vi "KI -Set Integral gain.vi"(1 "Action":bool, 3 "error in":errorcluster, 4 "Integral gain\nset":dbl format="%.2f", 5 "Axis #":i8=1 min=1 max=6 step=1, 6 "Address / Port":i16=1 min=1 max=31 step=1) -> (0 "error out":errorcluster, 2 "Integral gain\nread":string)   [LabVIEW 2014]
panel:
  # "Read"
  # "Write"
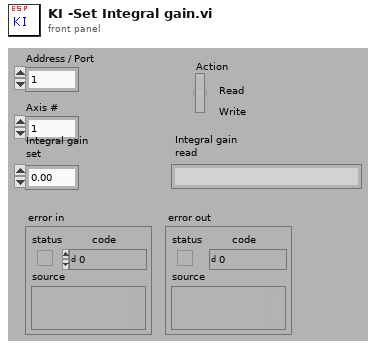
[diagram p1: front panel]
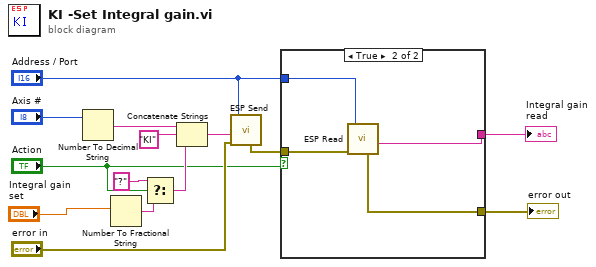
[diagram p0: block diagram]
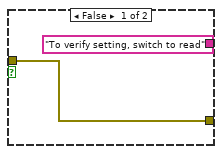
[diagram p2: hidden frame]
diagram:
  n1 = Number To Decimal String(number="Axis #") -> (decimal integer string=w13:string)  [unwired: 1 in]
  n2 = Number To Fractional String(number="Integral gain\nset") -> (F-format string=w9:string)  [unwired: 3 in]
  n3 = Select(t="?", s="Action", f=w9) -> (s? t:f=w10:string)
  n4 = Concatenate Strings(w13, "KI" ("Substring"), w10) -> (w11:string)
  n5 = call "ESP Send.vi"("Address / Port"="Address / Port", "Command String"=w11, "error in"="error in") -> ("error out"=w4:errorcluster)  [unwired: 5 in]
  n6 = case shown="True" "Action" {
    tunnel: "Address / Port" -> [_ w20]
    tunnel: w4 -> [w16 w19]
    tunnel: [w16 w18] -> w3
    tunnel: ["To verify setting, switch to read" w17] -> w1
    frame False {
    }
    frame True {
      n7 = call "ESP Read.vi"("Address / Port"=w20, "error in"=w19) -> ("error out"=w18:errorcluster, "Response String"=w17:string)  [unwired: 5 in]
    }
  }
  "error out" <- w3
  "Integral gain\nread" <- w1
